vi "Connect.vi"(8 "error in (no error)":errorcluster, 11 "Picomotor8742Comm in":refnum<class "TCPCommClass.lvclass">) -> (0 "error out":errorcluster, 3 "Picomotor8742Comm out":refnum<class "TCPCommClass.lvclass">)   [LabVIEW 2013, in "TCPCommClass.lvclass"]
uses:
  TCPCommClass.lvclass
  TCPCommClass.lvclass/TCPCommClass.ctl
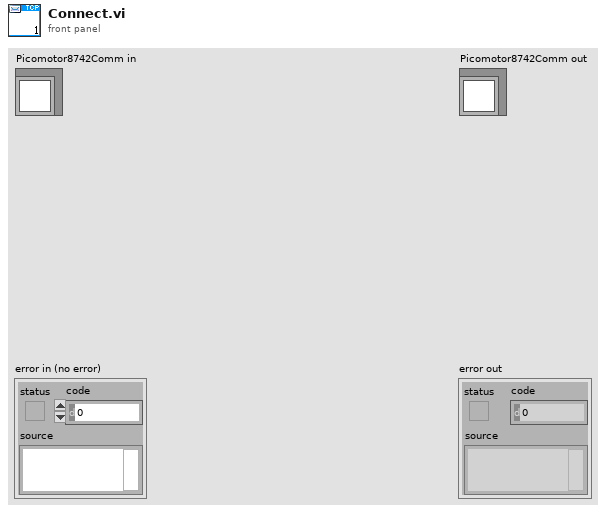
[diagram p1: front panel]
types:
  T1 = enum16{"Standard", "Buffered", "CRLF", "Immediate"}
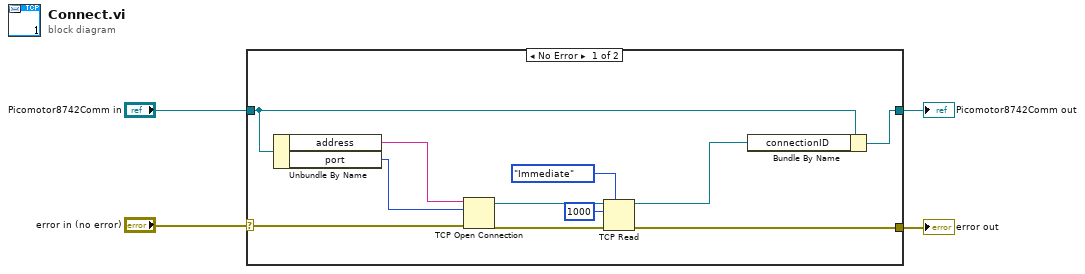
[diagram p0: block diagram]
diagram:
  n1 = case shown="No Error" "error in (no error)" {
    selector: "error in (no error)" -> [w11 w17]
    tunnel: [w7 w17] -> w3
    tunnel: [w6 w16] -> w1
    tunnel: "Picomotor8742Comm in" -> [w10 w16]
    frame No Error {
      n2 = Unbundle By Name(w10) -> ("address"=w9:string, "port"=w8:u16)
      n3 = TCP Open Connection(address=w9, remote port or service name=w8, error in (no error)=w11) -> (connection ID=w14:refnum<k5>, error out=w15:errorcluster)  [unwired: 2 in]
      n4 = TCP Read(connection ID=w14, bytes to read=1000, error in (no error)=w15, 7:T1."Immediate" ("mode (standard)")) -> (connection ID out=w5:refnum<k5>, error out=w7:errorcluster)  [unwired: 1 in, 1 out]
      n5 = Bundle By Name(cluster=w10, "connectionID"=w5) -> (w6:refnum<class "TCPCommClass.lvclass">)
    }
    frame Error {
    }
  }
  "error out" <- w3
  "Picomotor8742Comm out" <- w1
